vi "fromDevVarFloatArray.vi"(1 "argin":sgl[](array[numeric])) -> (0 "ArgIO":cluster{"num data":u8[], "str data":string[]})   [LabVIEW 2014, in "tango.lvlib"]
uses:
  tango.lvlib
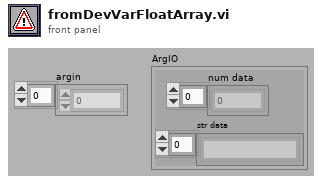
[diagram p1: front panel]
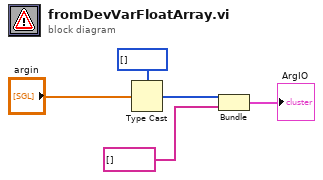
[diagram p0: block diagram]
diagram:
  n1 = Type Cast(type=u8[] [], x="argin") -> (*(type *) &x=w2:u8[])
  n2 = Bundle(w2, string[] []) -> (→"ArgIO":cluster{u8[], string[]})  [unwired: 1 in]
